vi "Send Message.vi"(8 "error in (no error)":errorcluster, 10 "TX Message":string="010C", 11 "PID in":refnum<class "PID.lvclass">) -> (0 "error out":errorcluster, 3 "PID out":refnum<class "PID.lvclass">)   [LabVIEW 2011, in "PID.lvclass"]
uses:
  PID.lvclass
  PID.lvclass/PID.ctl
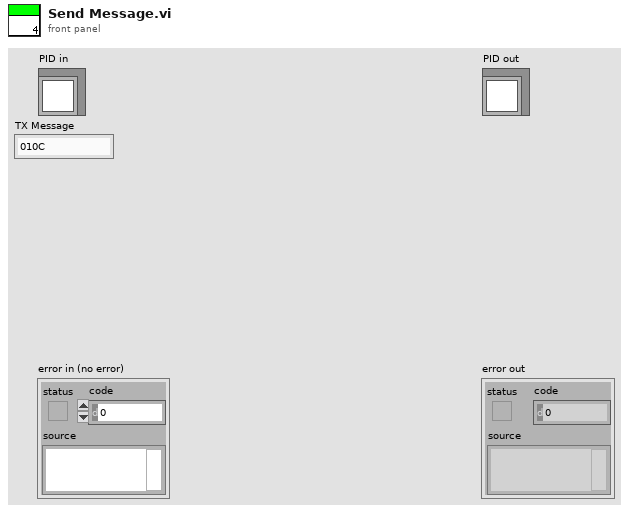
[diagram p1: front panel]
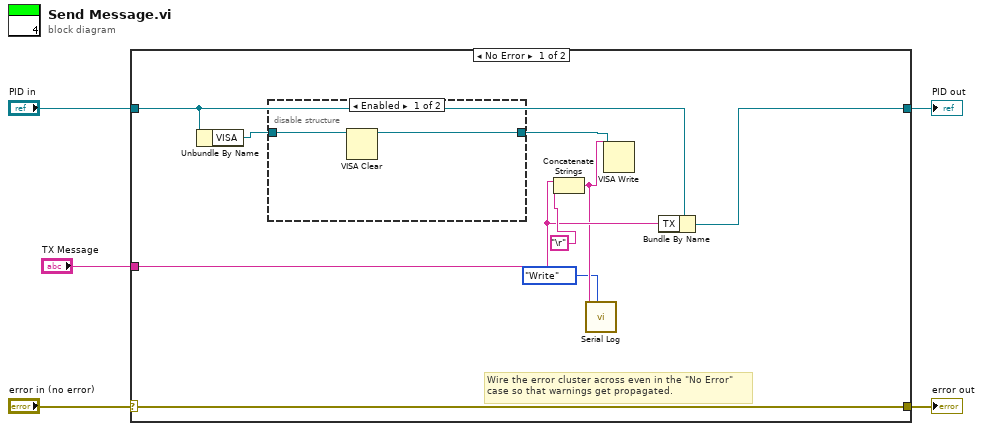
[diagram p0: block diagram]
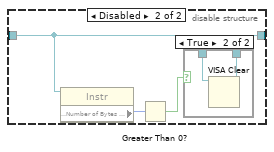
[diagram p2: hidden frame]
diagram:
  n1 = case shown="No Error" "error in (no error)" {
    selector: "error in (no error)" -> [w14 w25]
    tunnel: [w14 w25] -> w4
    tunnel: [w8 w24] -> w2
    tunnel: "PID in" -> [w9 w24]
    tunnel: "TX Message" -> [w10 _]
    frame No Error {
      # "Wire the error cluster across even in the \"No Error\"\ncase so that warnings get propagated."
      n2 = Unbundle By Name(w9) -> ("VISA"=w11:refnum<visa-resource-name>)
      n3 = disable-structure shown="Enabled" {
        disable-tunnel: [w16 w18] -> w12
        disable-tunnel: w11 -> [w15 w19]
        frame Enabled {
          n4 = VISA Clear(VISA resource name=w15) -> (VISA resource name out=w16:refnum<visa-resource-name>)  [unwired: 1 in, 1 out]
        }
        frame Disabled {
          n5 = property class="Instr"(reference=w19) -> ("Serial Settings:Number of Bytes at Serial Port"=w20:u32)  [unwired: 1 in, 2 out]
          n6 = Greater Than 0?(x=w20) -> (x > 0?=w17:bool)
          n7 = case shown="True" w17 {
            tunnel: w19 -> [w21 w23]
            tunnel: [w21 w22] -> w18
            frame False {
            }
            frame True {
              n8 = VISA Clear(VISA resource name=w23) -> (VISA resource name out=w22:refnum<visa-resource-name>)  [unwired: 1 in, 1 out]
            }
          }
        }
      }
      n9 = Concatenate Strings(w10, "\r") -> (w7:string)
      n10 = call "Serial Log.vi"("State"=enum16{"Init", "Write", "Read"}."Write", "String"=w7) -> ()  [unwired: 7 in, 3 out]
      n11 = VISA Write(VISA resource name=w12, write buffer=w7) -> ()  [unwired: 1 in, 3 out]
      n12 = Bundle By Name(cluster=w9, "TX"=w10) -> (w8:refnum<class "PID.lvclass">)
    }
    frame Error {
    }
  }
  "error out" <- w4
  "PID out" <- w2
